vi "Autonomous Independent.vi"() -> ()   [LabVIEW 2018]
doc: "This VI is called when autonomous begins, and will automatically be terminated when autonomous ends. You can carry out timed or sensor driven robot movement independently without needing to return to the caller."
uses:
  <vilib>/Rock Robotics/Network Tables/NT Read String.vi
  Robot Global Data.vi
  <vilib>/Rock Robotics/WPI/RobotDrive/WPI_RobotDriveArcadeDrive_Standard(NoSaturation).vi
  <vilib>/Rock Robotics/Network Tables/NT Write Numeric Array.vi
panel:
  in  "milliseconds to wait":u32=500
  in  "stage1downTime":u32=2000
  in  "stage2downTime":u32=250
  in  "rottionTime90":u32=1500
  out "Current Movement, for debugging":T1 {"Y Joystick Value" scale=1.0..-1.0; "X Joystick Value" scale=-1.0..1.0}
  in  "Array of robot movements":T2(array[cluster])=[{"X Joystick Value"=0.39393939393939403, "Y Joystick Value"=0.0, "Delay (sec)"=1.0, "Movement Name"="turn"}, {"X Joystick Value"=-0.3737373737373737, "Y Joystick Value"=0.0, "Delay (sec)"=1.0, "Movement Name"="turn back"}] {"Y Joystick Value" scale=1.0..-1.0; "X Joystick Value" scale=-1.0..1.0}
  # "Be sure to right-click and choose Data Operations>>Make Current Value default if you want to save the array values with the VI"
  # "Timeing for out of Start Position\nin Auto"
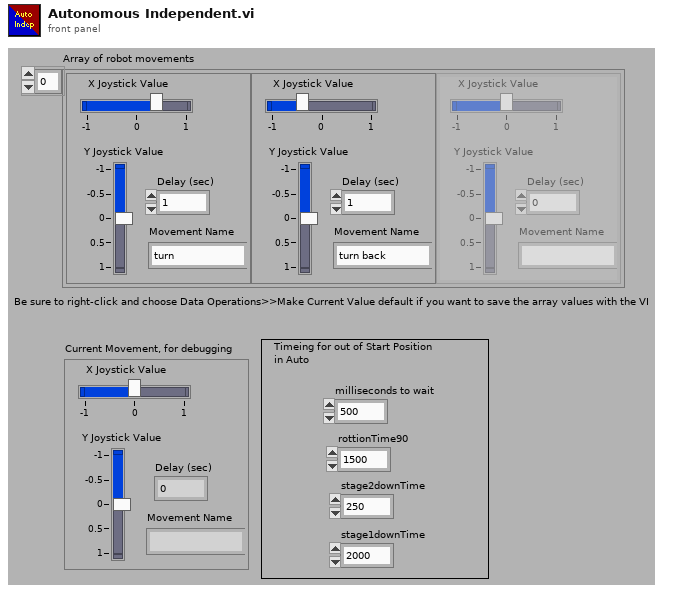
[diagram p1: front panel]
types:
  T1 = cluster{"X Joystick Value":dbl, "Y Joystick Value":dbl, "Delay (sec)":dbl, "Movement Name":string}
  T2 = cluster{"X Joystick Value":dbl, "Y Joystick Value":dbl, "Delay (sec)":dbl, "Movement Name":string}[]
  T3 = typedef "WPI_JoystickDevRef.ctl" = cluster{"Device":T4}
  T4 = typedef "WPI_JoystickDeviceEnum.ctl" = enum16{"USB 0", "USB 1", "USB 2", "USB 3", "USB 4", "USB 5"}
  T5 = typedef "WPI_RobotDriveDevRef.ctl" = cluster{"DevStatus":errorcluster, "Motors[]":T6[], "Square Inputs":bool, "Max Output":dbl}
  T6 = typedef "WPI_MotorControlDeviceRef.ctl" = cluster{"DeviceStatus":errorcluster, "Type":T7, "PWM":cluster{"PWM Channel":T8, "DeadBand":T9}, "CAN":cluster{"Device Number":u8, "SetOutput VI Ref":variant, "GetOutput VI Ref":variant, "Enable VI Ref":variant, "Disable VI Ref":variant, "Data":variant}, "Invert":bool, "DIO PWM":cluster{"PWM \"Enable\" Channel":T8, "DIOChannel":T10, "PWM Rate":dbl}}
  T7 = typedef "WPI_MotorControlType.ctl" = enum16{"PWM", "CAN", "DIO PWM"}
  T8 = typedef "FPGA_DIOPWMChannel.ctl" = enum8{"PWM 0", "PWM 1", "PWM 2", "PWM 3", "PWM 4", "PWM 5", "PWM 6", "PWM 7", "PWM 8", "PWM 9", "PWM MXP 0", "PWM MXP 1", "PWM MXP 2", "PWM MXP 3", "PWM MXP 4", "PWM MXP 5", "PWM MXP 6", "PWM MXP 7", "PWM MXP 8", "PWM MXP 9", "Invalid"}
  T9 = typedef "WPI_PWMDeadband.ctl" = cluster{"Name":string, "maxPositivePwm":i32, "minPositivePwm":i32, "centerPwm":i32, "maxNegativePwm":i32, "minNegativePwm":i32, "angularRange":u16}
  T10 = typedef "FPGA_DIOChannel.ctl" = enum8{"DIO 0", "DIO 1", "DIO 2", "DIO 3", "DIO 4", "DIO 5", "DIO 6", "DIO 7", "DIO 8", "DIO 9", "DIO MXP 0", "DIO MXP 1", "DIO MXP 2", "DIO MXP 3", "DIO MXP 4", "DIO MXP 5", "DIO MXP 6", "DIO MXP 7", "DIO MXP 8", "DIO MXP 9", "DIO MXP 10", "DIO MXP 11", "DIO MXP 12", "DIO MXP 13", "DIO MXP 14", "DIO MXP 15", "SPI Port CS1", "SPI Port CS2", "SPI Port CS3", "SPI Port MISO", "SPI Port MOSI", "Invalid"}
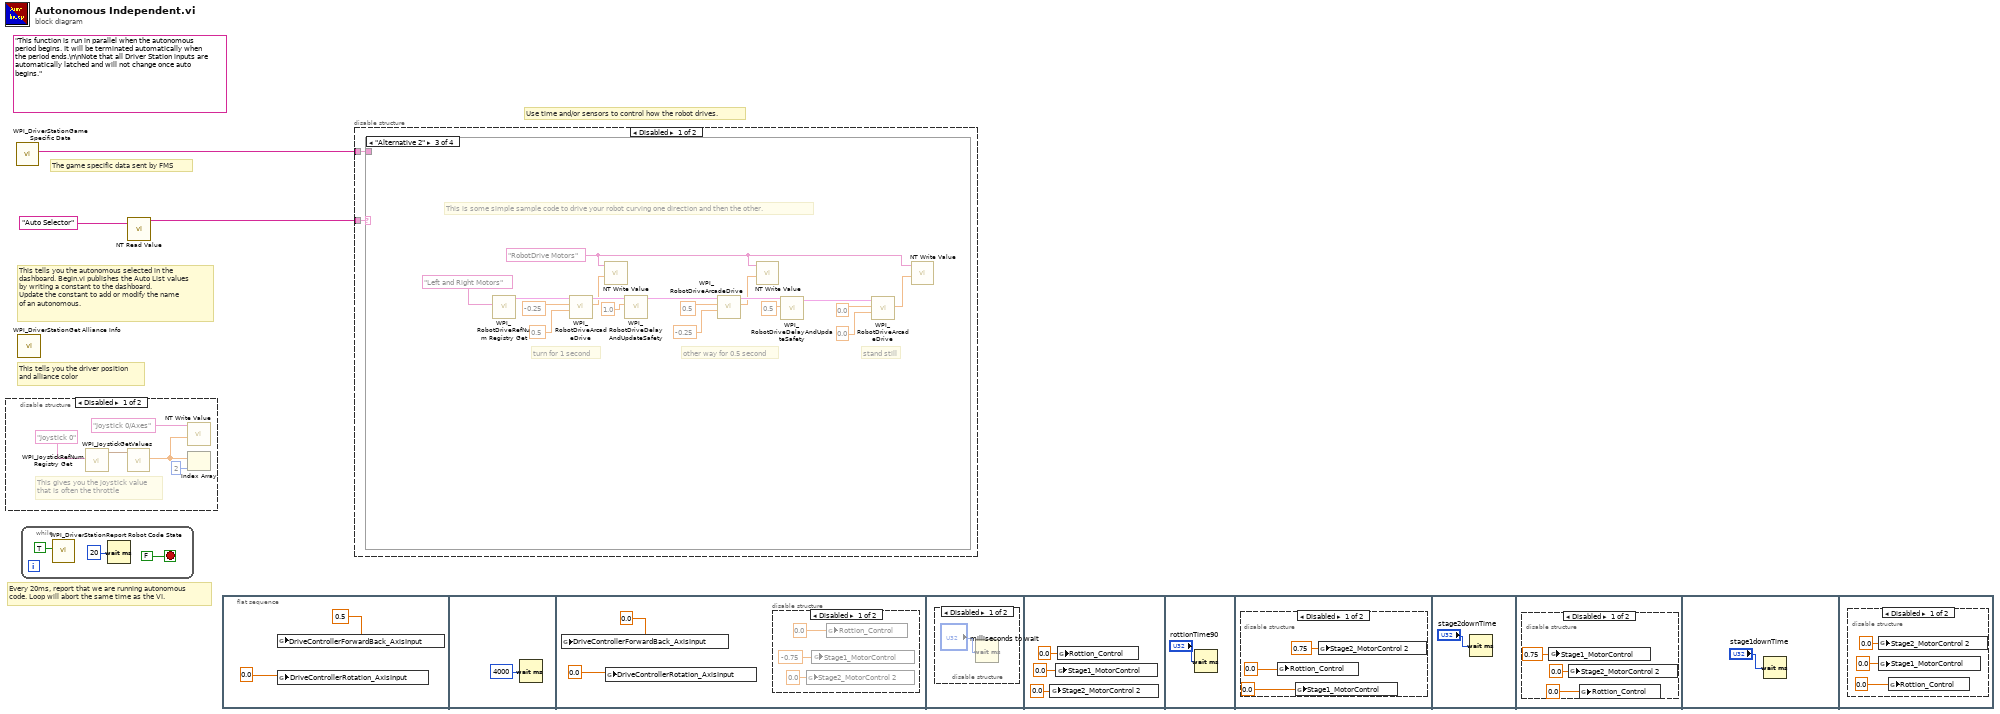
[diagram p0: block diagram]
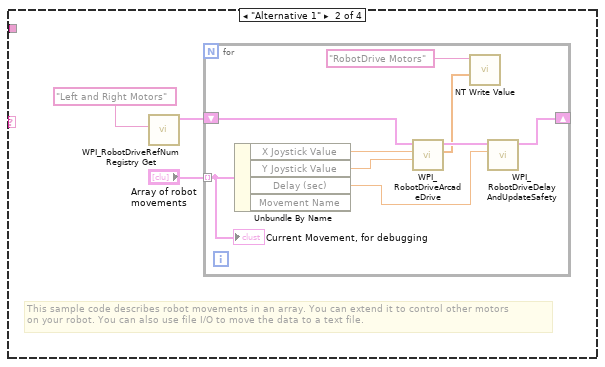
[diagram p9: hidden frame]
diagram:
  (unwired) "This function is run in parallel when the autonomous period begins. It will be terminated automatically when the period ends.\n\nNote that all Driver Station inputs are automatically latched and will not change once auto begins."
  # "The game specific data sent by FMS"
  # "This tells you the autonomous selected in the \ndashboard. Begin.vi publishes the Auto List values\nby writing a constant to the dashboard.\nUpdate the constant to add or modify the name\nof an autonomous."
  # "Every 20ms, report that we are running autonomous\ncode. Loop will abort the same time as the VI."
  # "Use time and/or sensors to control how the robot drives."
  # "This tells you the driver position\nand alliance color"
  n1 = disable-structure shown="Disabled" {
    frame Disabled {
      # "This gives you the joystick value\nthat is often the throttle"
      n2 = call <vilib>:"WPI_JoystickRefNum Registry Get.vi"("refnum name"="Joystick 0") -> ("JoystickDevRef"=w7:T3)  [unwired: 1 in, 9 out]
      n3 = call <vilib>:"WPI_JoystickGetValues.vi"("JoystickDevRef"=w7) -> ("Axes"=w5:dbl[])  [unwired: 6 in, 4 out]
      n4 = call-poly <vilib>:"NT Write Value.vi"("Numeric Array"=w5, "Name"="Joystick 0/Axes") -> ()  [unwired: 9 in, 1 out]
      n5 = Index Array(array=w5, index=2) -> ()  [unwired: 1 out]
    }
    frame Enabled {
    }
  }
  n6 = call <vilib>:"WPI_DriverStationGame Specific Data.vi"() -> ("Game Specific Data"=w1:string)  [unwired: 11 in]
  n7 = call <vilib>:"WPI_DriverStationGet Alliance Info.vi"() -> ()  [unwired: 12 out]
  n8 = while {
    stop <- FALSE stop-if-true
    n9 = call <vilib>:"WPI_DriverStationReport Robot Code State.vi"("Autonomous"=TRUE) -> ()  [unwired: 10 in, 1 out]
    n10 = Wait (ms)(milliseconds to wait=u32 20) -> ()  [unwired: 1 out]
  }
  n11 = call-poly <vilib>:"NT Read Value.vi"("Name"="Auto Selector") -> ("String"=w2:string)  [unwired: 9 in, 1 out]
  n12 = flat-sequence {
    frame #0 {
      n13 = global write "Robot Global Data.vi" "DriveControllerForwardBack_AxisInput"(0.5 ("X axis value")) -> ()
      n14 = global write "Robot Global Data.vi" "DriveControllerRotation_AxisInput"(0.0 ("DriveControllerRotation_AxisInput")) -> ()
    }
    frame #1 {
      n15 = Wait (ms)(milliseconds to wait=u32 4000) -> ()  [unwired: 1 out]
    }
    frame #2 {
      n16 = global write "Robot Global Data.vi" "DriveControllerForwardBack_AxisInput"(0.0 ("X axis value")) -> ()
      n17 = global write "Robot Global Data.vi" "DriveControllerRotation_AxisInput"(0.0 ("X axis value")) -> ()
      n18 = disable-structure shown="Disabled" {
        frame Disabled {
          n19 = global write "Robot Global Data.vi" "Stage2_MotorControl 2"(0.0 ("Stage2_MotorControl 2")) -> ()
          n20 = global write "Robot Global Data.vi" "Stage1_MotorControl"(-0.75 ("Stage2_MotorControl 2")) -> ()
          n21 = global write "Robot Global Data.vi" "Rottion_Control"(0.0 ("Stage2_MotorControl 2")) -> ()
        }
        frame Enabled {
        }
      }
    }
    frame #3 {
      n22 = disable-structure shown="Disabled" {
        frame Disabled {
          n23 = Wait (ms)(milliseconds to wait="milliseconds to wait") -> ()  [unwired: 1 out]
        }
        frame Enabled {
        }
      }
    }
    frame #4 {
      n24 = global write "Robot Global Data.vi" "Stage2_MotorControl 2"(0.0 ("Stage2_MotorControl 2")) -> ()
      n25 = global write "Robot Global Data.vi" "Stage1_MotorControl"(0.0 ("Stage2_MotorControl 2")) -> ()
      n26 = global write "Robot Global Data.vi" "Rottion_Control"(0.0 ("Rottion_Control")) -> ()
    }
    frame #5 {
      n27 = Wait (ms)(milliseconds to wait="rottionTime90") -> ()  [unwired: 1 out]
    }
    frame #6 {
      n28 = disable-structure shown="Disabled" {
        frame Disabled {
          n29 = global write "Robot Global Data.vi" "Rottion_Control"(0.0 ("Stage2_MotorControl 2")) -> ()
          n30 = global write "Robot Global Data.vi" "Stage1_MotorControl"(0.0 ("Stage2_MotorControl 2")) -> ()
          n31 = global write "Robot Global Data.vi" "Stage2_MotorControl 2"(0.75 ("Stage2_MotorControl 2")) -> ()
        }
        frame Enabled {
        }
      }
    }
    frame #7 {
      n32 = Wait (ms)(milliseconds to wait="stage2downTime") -> ()  [unwired: 1 out]
    }
    frame #8 {
      n33 = disable-structure shown="Disabled" {
        frame Disabled {
          n34 = global write "Robot Global Data.vi" "Stage1_MotorControl"(0.75 ("Stage1_MotorControl")) -> ()
          n35 = global write "Robot Global Data.vi" "Stage2_MotorControl 2"(0.0 ("Stage2_MotorControl 2")) -> ()
          n36 = global write "Robot Global Data.vi" "Rottion_Control"(0.0 ("Stage2_MotorControl 2")) -> ()
        }
        frame Enabled {
        }
      }
    }
    frame #9 {
      n37 = Wait (ms)(milliseconds to wait="stage1downTime") -> ()  [unwired: 1 out]
    }
    frame #10 {
      n38 = disable-structure shown="Disabled" {
        frame Disabled {
          n39 = global write "Robot Global Data.vi" "Stage2_MotorControl 2"(0.0 ("Stage2_MotorControl 2")) -> ()
          n40 = global write "Robot Global Data.vi" "Stage1_MotorControl"(0.0 ("Stage2_MotorControl 2")) -> ()
          n41 = global write "Robot Global Data.vi" "Rottion_Control"(0.0 ("Stage2_MotorControl 2")) -> ()
        }
        frame Enabled {
        }
      }
    }
  }
  n42 = disable-structure shown="Disabled" {
    disable-tunnel: w2 -> [w37 _]
    disable-tunnel: w1 -> [w36 _]
    frame Disabled {
      n43 = case shown="\"Alternative 2\"" w37 {
        tunnel: w36 -> [_ _ _ _]
        frame Default {
          # "You can put your main auto here, or you can right-click on the case and make any\nother frame be the default case."
          # "This is the frame that will execute if no selection is made, or if it is not recognized"
        }
        frame "Alternative 1" {
          # "This sample code describes robot movements in an array. You can extend it to control other motors\non your robot. You can also use file I/O to move the data to a text file."
          n44 = call <vilib>:"WPI_RobotDriveRefNum Registry Get.vi"("refnum name"="Left and Right Motors") -> ("RobotDriveDevRef"=w39:T5)  [unwired: 1 in, 9 out]
          n45 = for {
            shift-right: [w47] -> _
            shift-left: w39 -> [w48]
            tunnel: "Array of robot movements" -> [w43] mode=indexing
            n46 = Unbundle By Name(w43) -> ("X Joystick Value"=w46:dbl, "Y Joystick Value"=w45:dbl, "Delay (sec)"=w44:dbl)  [unwired: 1 out]
            n47 = call-poly <vilib>:"WPI_RobotDriveArcadeDrive.vi"("Y axis value"=w45, "X axis value"=w46, "RobotDriveDevRef"=w48) -> ("Motor Values"=w41:dbl[], "RobotDriveDevRef"=w49:T5)  [unwired: 1 in, 6 out]
            n48 = call-poly <vilib>:"NT Write Value.vi"("Numeric Array"=w41, "Name"="RobotDrive Motors") -> ()  [unwired: 9 in, 1 out]
            n49 = call <vilib>:"WPI_RobotDriveDelayAndUpdateSafety.vi"("Delay (s)"=w44, "RobotDriveDevRef"=w49) -> ("RobotDriveDevRef 2"=w47:T5)  [unwired: 8 in, 1 out]
            "Current Movement, for debugging" <- w43
          }
        }
        frame "Alternative 2" {
          w51 = "RobotDrive Motors" ("Name")
          # "This is some simple sample code to drive your robot curving one direction and then the other."
          # "stand still"
          # "other way for 0.5 second"
          # "turn for 1 second"
          n50 = call <vilib>:"WPI_RobotDriveRefNum Registry Get.vi"("refnum name"="Left and Right Motors") -> ("RobotDriveDevRef"=w67:T5)  [unwired: 1 in, 9 out]
          n51 = call-poly <vilib>:"WPI_RobotDriveArcadeDrive.vi"("Y axis value"=0.5 ("X axis value"), "X axis value"=-0.25, "RobotDriveDevRef"=w67) -> ("Motor Values"=w50:dbl[], "RobotDriveDevRef"=w60:T5)  [unwired: 1 in, 6 out]
          n52 = call-poly <vilib>:"NT Write Value.vi"("Numeric Array"=w50, "Name"=w51) -> ()  [unwired: 9 in, 1 out]
          n53 = call <vilib>:"WPI_RobotDriveDelayAndUpdateSafety.vi"("Delay (s)"=1.0, "RobotDriveDevRef"=w60) -> ("RobotDriveDevRef 2"=w61:T5)  [unwired: 8 in, 1 out]
          n54 = call-poly <vilib>:"WPI_RobotDriveArcadeDrive.vi"("Y axis value"=-0.25 ("X axis value"), "X axis value"=0.5, "RobotDriveDevRef"=w61) -> ("Motor Values"=w52:dbl[], "RobotDriveDevRef"=w62:T5)  [unwired: 1 in, 6 out]
          n55 = call-poly <vilib>:"NT Write Value.vi"("Numeric Array"=w52, "Name"=w51) -> ()  [unwired: 9 in, 1 out]
          n56 = call <vilib>:"WPI_RobotDriveDelayAndUpdateSafety.vi"("Delay (s)"=0.5, "RobotDriveDevRef"=w62) -> ("RobotDriveDevRef 2"=w63:T5)  [unwired: 8 in, 1 out]
          n57 = call-poly <vilib>:"WPI_RobotDriveArcadeDrive.vi"("Y axis value"=0.0 ("X axis value"), "X axis value"=0.0, "RobotDriveDevRef"=w63) -> ("Motor Values"=w53:dbl[])  [unwired: 1 in, 7 out]
          n58 = call-poly <vilib>:"NT Write Value.vi"("Numeric Array"=w53, "Name"=w51) -> ()  [unwired: 9 in, 1 out]
        }
        frame "Your Turn" {
        }
      }
    }
    frame Enabled {
    }
  }
